vi "CreateOverrides.vi"(8 "error in (no error)":errorcluster, 11 "CreateClass in":refnum<class "CreateClass.lvclass">) -> (0 "error out":errorcluster, 3 "CreateClass out":refnum<class "CreateClass.lvclass">)   [LabVIEW 2020, in "Mermaid.lvlib" / "CreateClass.lvclass"]
uses:
  CreateClass.lvclass
  CreateClass.lvclass/CreateClass.ctl
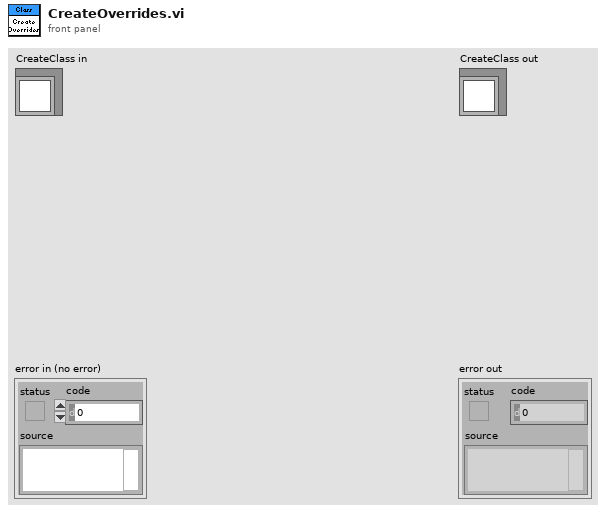
[diagram p1: front panel]
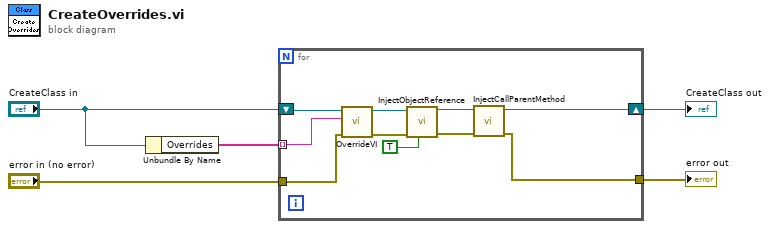
[diagram p0: block diagram]
diagram:
  n1 = Unbundle By Name("CreateClass in") -> ("Overrides"=w5:string[])
  n2 = for {
    tunnel: w5 -> [w14] mode=indexing
    tunnel: "error in (no error)" -> [w13]
    shift-right: [w6] -> w2
    shift-left: "CreateClass in" -> [w15]
    tunnel: [w7] -> w1
    n3 = call "OverrideVI.vi"("error in (no error)"=w13, "Name"=w14, "CreateClass In"=w15) -> ("error out"=w11:errorcluster, "CreateClass Out"=w12:refnum<class "CreateClass.lvclass">)  [unwired: 7 in]
    n4 = call "InjectObjectReference.vi"("Dynamic Dispatch"=TRUE, "error in (no error)"=w11, "CreateClass In"=w12) -> ("error out"=w8:errorcluster, "CreateClass Out"=w9:refnum<class "CreateClass.lvclass">)  [unwired: 7 in]
    n5 = call "InjectCallParentMethod.vi"("error in (no error)"=w8, "CreateClass in"=w9) -> ("error out"=w7:errorcluster, "CreateClass out"=w6:refnum<class "CreateClass.lvclass">)  [unwired: 8 in]
  }
  "error out" <- w1
  "CreateClass out" <- w2
